vi "Set Automatic Exposure Mode.vi.vi"(8 "error in (no error)":errorcluster, 10 "Automatic Parameter Mode":T1, 11 "Stream":refnum<data-value>) -> (0 "error out":errorcluster, 3 "Stream (duplicate)":refnum<data-value>)   [LabVIEW 2020, in "g_ar_toolkit.capture.lvlib" / "CameraStream.lvclass"]
uses:
  CameraStream.lvclass
  CameraStream.lvclass/CameraStream.ctl
  Camera Automatic Parameters.ctl
  Camera Automatic Parameter Mode.ctl
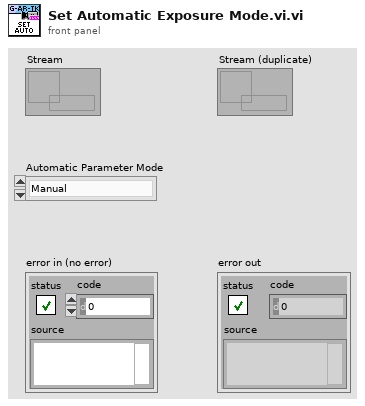
[diagram p1: front panel]
types:
  T1 = typedef "g_ar_toolkit.capture.lvlib/CameraStream.lvclass/Camera Automatic Parameter Mode.ctl" = enum16{"Manual", "Automatic"}
  T2 = typedef "g_ar_toolkit.capture.lvlib/CameraStream.lvclass/Camera Automatic Parameters.ctl" = enum16{"AUTO_EXPOSURE", "AUTO_FOCUS", "AUTO_WHITEBALANCE", "AUTO_GAIN"}
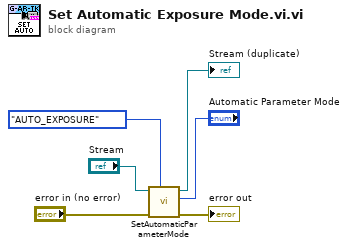
[diagram p0: block diagram]
diagram:
  n1 = call "SetAutomaticParameterMode.vi"("Auto Parameter"=Camera_Automatic_Parameters."AUTO_EXPOSURE", "error in (no error)"="error in (no error)", "Automatic"="Automatic Parameter Mode", "Stream"="Stream") -> ("error out"=→"error out":errorcluster, "Stream (duplicate)"=→"Stream (duplicate)":refnum<data-value>)  [unwired: 6 in]
